vi "Configure Measurement (Multi-Carrier Power).vi"(0 "VISA resource name":refnum<visa-resource-name>, 1 "Enable Limit Test (F: Disable)":bool, 2 "Enable Noise Correction (F: Disable)":bool, 5 "Enable Auto Power Reference (T: Enable)":bool=TRUE, 7 "Manual Power Reference (10)":dbl=10.0 format="%#.6g", 9 "Method":u16(ring) items=["Integration Bandwidth", "Resolution Bandwidth"], 11 "error in (no error)":errorcluster) -> (4 "VISA resource name out":refnum<visa-resource-name>, 15 "error out":errorcluster)   [LabVIEW 2014, in "Agilent ESA PSA Series.lvlib"]
doc: "Sets up the multi carrier power measurement."
uses:
  Agilent ESA PSA Series.lvlib
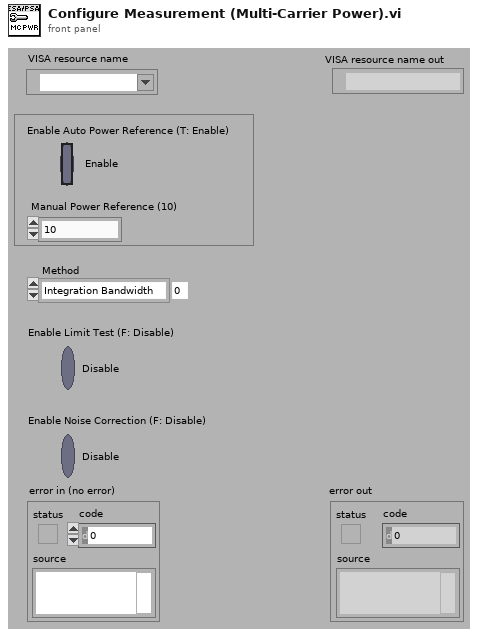
[diagram p1: front panel]
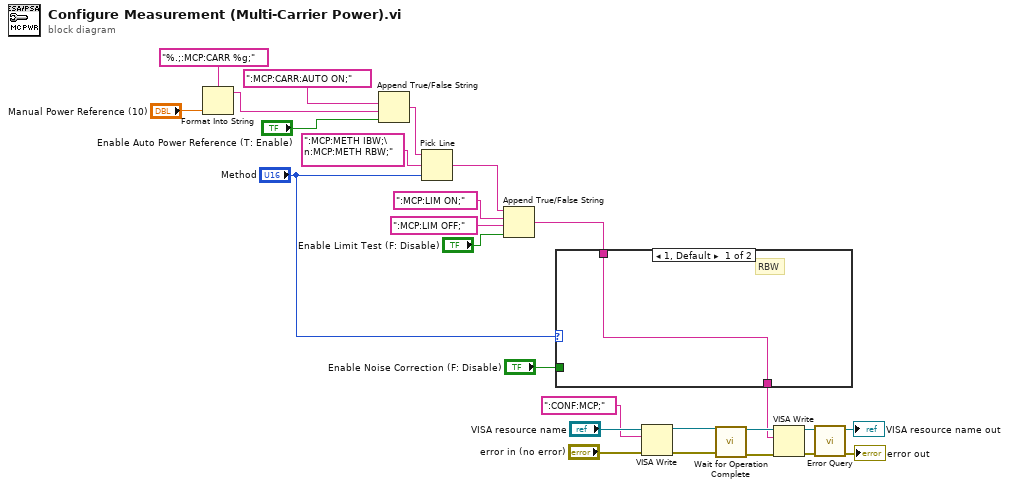
[diagram p0: block diagram]
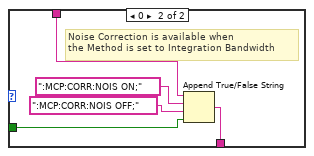
[diagram p2: hidden frame]
diagram:
  n1 = Format Into String(format string="%.;:MCP:CARR %g;", "Manual Power Reference (10)") -> (resulting string=w5:string)  [unwired: 2 in, 1 out]
  n2 = Append True/False String(1:"Enable Auto Power Reference (T: Enable)", 2:w5, 3:":MCP:CARR:AUTO ON;" ("initial string")) -> (0:w3:string)  [unwired: 1 in]
  n3 = Pick Line(string ("")=w3, multi-line string=":MCP:METH IBW;\n:MCP:METH RBW;" ("false string"), line index="Method") -> (output string=w2:string)
  n4 = Append True/False String(1:"Enable Limit Test (F: Disable)", 2:":MCP:LIM OFF;" ("false string"), 3:":MCP:LIM ON;" ("false string"), 4:w2) -> (0:w1:string)
  n5 = case shown="1, Default" "Method" {
    tunnel: w1 -> [w27 w30]
    tunnel: "Enable Noise Correction (F: Disable)" -> [_ w29]
    tunnel: [w27 w28] -> w4
    frame 1, Default {
      # "RBW"
    }
    frame 0 {
      # "Noise Correction is available when\nthe Method is set to Integration Bandwidth"
      n6 = Append True/False String(1:w29, 2:":MCP:CORR:NOIS OFF;" ("false string"), 3:":MCP:CORR:NOIS ON;" ("false string"), 4:w30) -> (0:w28:string)
    }
  }
  n7 = VISA Write(VISA resource name="VISA resource name", write buffer=":CONF:MCP;" ("initial string"), error in (no error)="error in (no error)") -> (VISA resource name out=w9:refnum<visa-resource-name>, error out=w10:errorcluster)  [unwired: 1 out]
  n8 = call "Wait for Operation Complete.vi"("error in (no error)"=w10, "VISA resource name"=w9) -> ("error out"=w13:errorcluster, "VISA resource name out"=w14:refnum<visa-resource-name>)  [unwired: 8 in]
  n9 = VISA Write(VISA resource name=w14, write buffer=w4, error in (no error)=w13) -> (VISA resource name out=w16:refnum<visa-resource-name>, error out=w15:errorcluster)  [unwired: 1 out]
  n10 = call "Error Query.vi"("error in (no error)"=w15, "VISA resource name"=w16) -> ("error out"=→"error out":errorcluster, "VISA resource name out"=→"VISA resource name out":refnum<visa-resource-name>)  [unwired: 6 in, 2 out]
